vi "Untitled 1 (SubVI).vi"(11 "Numeric in":i32) -> (3 "Numeric out":i32)   [LabVIEW 2017]
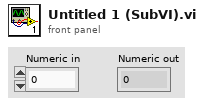
[diagram p1: front panel]
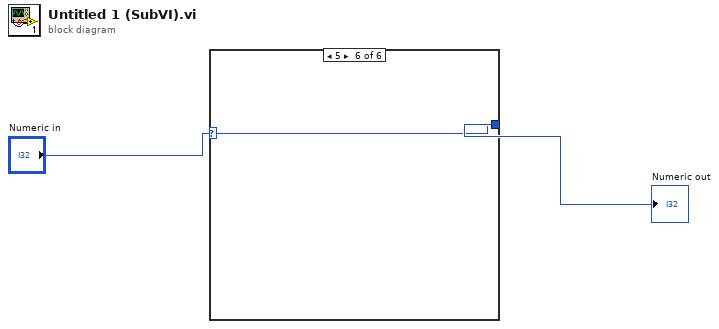
[diagram p0: block diagram]
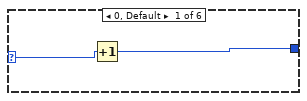
[diagram p2: hidden frame]
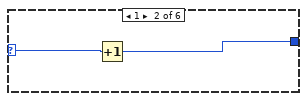
[diagram p3: hidden frame]
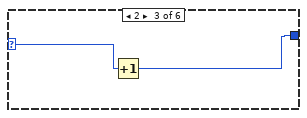
[diagram p4: hidden frame]
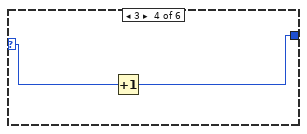
[diagram p5: hidden frame]
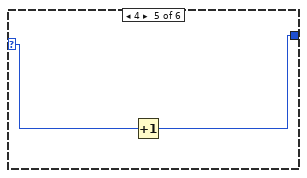
[diagram p6: hidden frame]
diagram:
  n1 = case shown="5" "Numeric in" {
    selector: "Numeric in" -> [w4 w6 w8 w10 w12 w13]
    tunnel: [w3 w5 w7 w9 w11 w13] -> w2
    frame 0, Default {
      n2 = Increment(x=w4) -> (x+1=w3:i32)
    }
    frame 1 {
      n3 = Increment(x=w6) -> (x+1=w5:i32)
    }
    frame 2 {
      n4 = Increment(x=w8) -> (x+1=w7:i32)
    }
    frame 3 {
      n5 = Increment(x=w10) -> (x+1=w9:i32)
    }
    frame 4 {
      n6 = Increment(x=w12) -> (x+1=w11:i32)
    }
    frame 5 {
    }
  }
  "Numeric out" <- w2
